vi "Open and Edit Error File.vi"() -> ()   [LabVIEW 2016, in "Error File Management.lvlib"]
uses:
  Error File Management.lvlib
  <vilib>/xml/NI_XML.lvlib
  <vilib>/xml/Close Reference(Node).vi
  <vilib>/xml/Load XML File.vi
  Controls/NI Family.ctl
  Controls/NI Error.ctl
panel:
  out "errors":T1[](array[typedef])
  out "comment":string
  out "family":T2
  out "error out":errorcluster
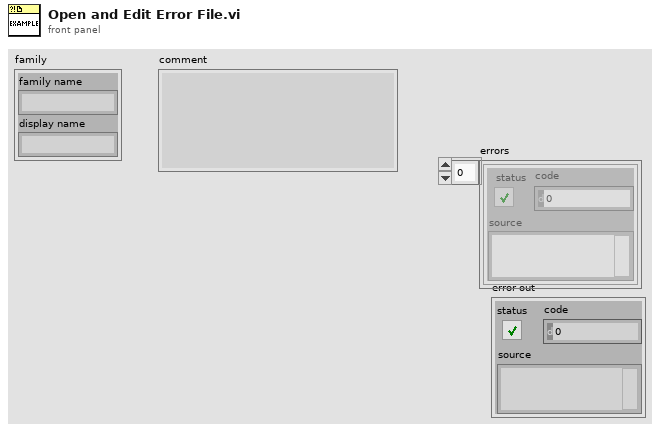
[diagram p1: front panel]
types:
  T1 = typedef "Error File Management.lvlib/NI Error.ctl" = errorcluster
  T2 = typedef "Error File Management.lvlib/NI Family.ctl" = cluster{"family name":string, "display name":string}
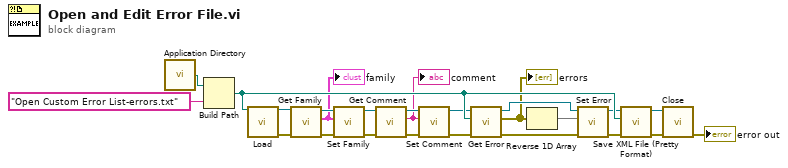
[diagram p0: block diagram]
diagram:
  n1 = call <vilib>:"Application Directory.vi"() -> ("Application Directory"=w3:path)
  n2 = Build Path(base path=w3, name or relative path="Open Custom Error List-errors.txt") -> (appended path=w24:path)
  n3 = call-poly <vilib>:"Load.vi"("path to XML document"=w24) -> ("DOM document out"=w23:refnum<k20>, "error out"=w22:errorcluster)  [unwired: 12 in, 1 out]
  n4 = call "Get Family.vi"("error in (no error)"=w22, "DOM document in"=w23) -> ("error out"=w21:errorcluster, "family"=w16:T2, "DOM document out"=w18:refnum<k20>)  [unwired: 7 in]
  "family" <- w16
  n5 = call "Set Family.vi"("error in (no error)"=w21, "family"=w16, "DOM document in"=w18) -> ("error out"=w19:errorcluster, "DOM document out"=w17:refnum<k20>)  [unwired: 7 in]
  n6 = call "Get Comment.vi"("error in (no error)"=w19, "DOM document in"=w17) -> ("error out"=w20:errorcluster, "comment"=w12:string, "DOM document out"=w14:refnum<k20>)  [unwired: 7 in]
  "comment" <- w12
  n7 = call "Set Comment.vi"("error in (no error)"=w20, "comment"=w12, "DOM document in"=w14) -> ("error out"=w15:errorcluster, "DOM document out"=w13:refnum<k20>)  [unwired: 7 in]
  n8 = call "Get Error.vi"("error in (no error)"=w15, 10:w24, "DOM document in"=w13) -> ("error out"=w6:errorcluster, "errors"=w1:T1[], "DOM document out"=w7:refnum<k20>)  [unwired: 6 in]
  "errors" <- w1
  n9 = Reverse 1D Array(array=w1) -> (reversed array=w8:T1[])
  n10 = call "Set Error.vi"("error in (no error)"=w6, "errors"=w8, "DOM document in"=w7) -> ("error out"=w5:errorcluster, "DOM document out"=w4:refnum<k20>)  [unwired: 7 in]
  n11 = call "Save XML File (Pretty Format).vi"("error in (no error)"=w5, "XML file path"=w24, "DOM document in"=w4) -> ("error out"=w11:errorcluster, "DOM document out"=w10:refnum<k20>)  [unwired: 6 in, 1 out]
  n12 = call-poly <vilib>:"Close.vi"("error in (no error)"=w11, "node"=w10) -> ("error out"=→"error out":errorcluster)  [unwired: 7 in]
